vi "Query Waveform Completed.vi"   [LabVIEW 2018, in "Agilent PSG MXG Series.lvlib"]
doc: "Query whether the ARB waveform has completed for Dual or Digital Modulation personalities."
uses:
  Agilent PSG MXG Series.lvlib
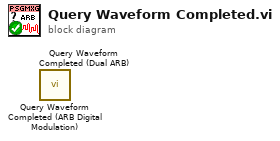
[diagram p0: block diagram]
diagram:
  n1 = call "Query Waveform Completed (ARB Digital Modulation).vi"() -> ()  [unwired: 9 in, 3 out]
  n2 = call "Query Waveform Completed (Dual ARB).vi"() -> ()  [unwired: 9 in, 3 out]
